vi "LWXPS_TestTCP.vi"(0 "XPS Reference IN":refnum<k24>, 7 "Input String":string, 11 "LabVIEW error IN":errorcluster) -> (4 "XPS Reference OUT":refnum<k24>, 6 "Returned error code":i32, 8 "Return String":string, 10 "XPS Error String":string, 15 "LabVIEW error OUT":errorcluster)   [LabVIEW 2014]
uses:
  D:/XPSQ8_LabView_Library/Development/Source/Dll/Newport.XPS.CommandInterface.dll
  Dll/Newport.XPS.CommandInterface.dll
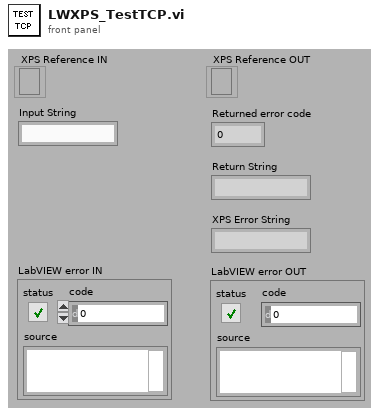
[diagram p1: front panel]
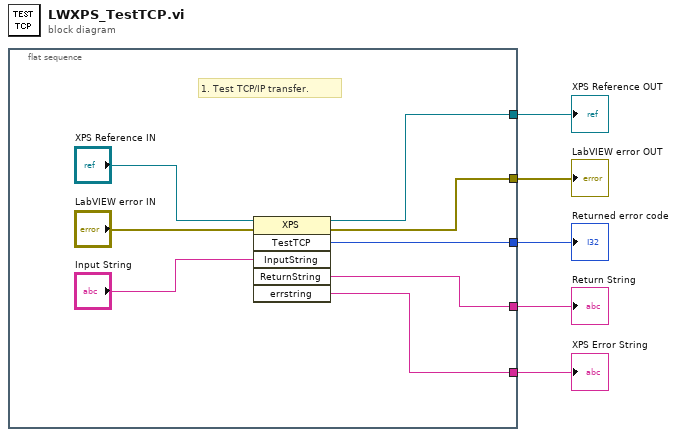
[diagram p0: block diagram]
diagram:
  n1 = flat-sequence {
    tunnel: [w11] -> w5
    tunnel: [w8] -> w4
    tunnel: [w12] -> w3
    tunnel: [w6] -> w1
    tunnel: [w7] -> w2
    frame #0 {
      # "1. Test TCP/IP transfer."
      n2 = invoke class="XPS" method="TestTCP"(reference="XPS Reference IN", error in="LabVIEW error IN", "InputString"="Input String") -> (reference out=w11:refnum<k24>, error out=w8:errorcluster, "TestTCP"=w12:i32, "ReturnString"=w6:string, "errstring"=w7:string)  [unwired: 3 in, 1 out]
    }
  }
  "XPS Error String" <- w2
  "XPS Reference OUT" <- w5
  "LabVIEW error OUT" <- w4
  "Returned error code" <- w3
  "Return String" <- w1
